vi "create_opti_path.vi"(2 "RunNumber":u16, 4 "base path":path) -> (0 "Path":path)   [LabVIEW 2020]
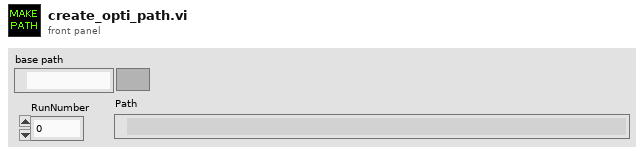
[diagram p1: front panel]
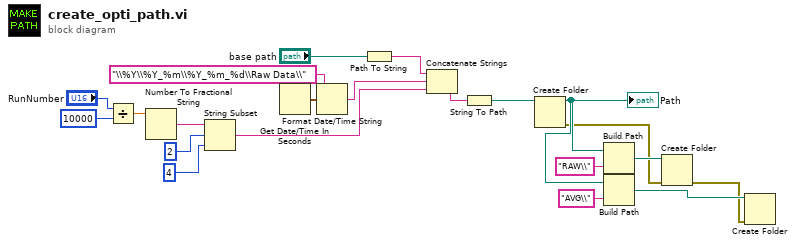
[diagram p0: block diagram]
diagram:
  n1 = Divide(x="RunNumber", y=u16 10000) -> (x/y=w16:dbl)
  n2 = Number To Fractional String(number=w16) -> (F-format string=w15:string)  [unwired: 3 in]
  n3 = String Subset(string=w15, offset (0)=2, length (rest)=4 ("length (rest)")) -> (substring=w12:string)
  n4 = Get Date/Time In Seconds() -> (seconds since 1Jan1904=w20:timestamp)
  n5 = Format Date/Time String(time format string (%c)="\\%Y\\%Y_%m\\%Y_%m_%d\\Raw Data\\", seconds (now)=w20) -> (date/time string=w19:string)  [unwired: 1 in]
  n6 = Path To String(path="base path") -> (string=w10:string)
  n7 = Concatenate Strings(w10, w19, w12) -> (w9:string)
  n8 = String To Path(string=w9) -> (path=w8:path)
  n9 = Create Folder(path (use dialog)=w8) -> (created path=w3:path, error out=w2:errorcluster)  [unwired: 2 in, 1 out]
  "Path" <- w3
  n10 = Build Path(base path=w3, name or relative path="RAW\\") -> (appended path=w5:path)
  n11 = Build Path(base path=w3, name or relative path="AVG\\") -> (appended path=w4:path)
  n12 = Create Folder(path (use dialog)=w5, error in=w2) -> (error out=w1:errorcluster)  [unwired: 1 in, 2 out]
  n13 = Create Folder(path (use dialog)=w4, error in=w1) -> ()  [unwired: 1 in, 3 out]
